vi "Write Rectifier Recipe to ListBox.vi"(4 "Right AmpMins":dbl[](array[numeric]), 5 "Left AmpMins":dbl[](array[numeric]), 6 "Right Amps":dbl[](array[numeric]), 7 "Left Amps":dbl[](array[numeric]), 8 "error in (no error)":errorcluster, 10 "Number Steps":i32, 11 "ListBox":refnum<vi>) -> (0 "error out":errorcluster)   [LabVIEW 2019]
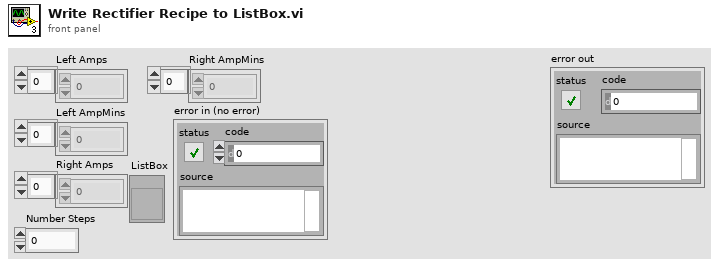
[diagram p1: front panel]
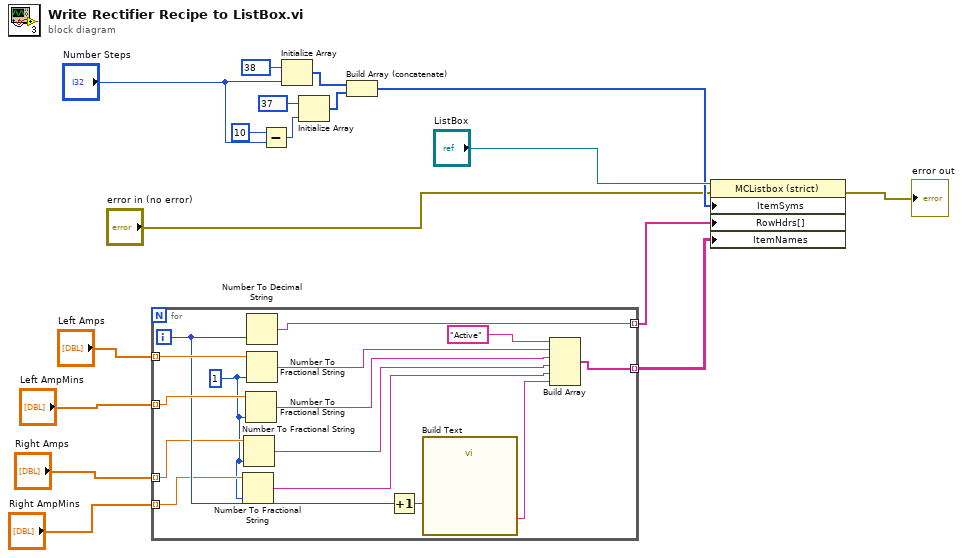
[diagram p0: block diagram]
diagram:
  n1 = for {
    tunnel: [w32] -> w2 mode=indexing
    tunnel: "Left Amps" -> [w29] mode=indexing
    tunnel: "Left AmpMins" -> [w26] mode=indexing
    tunnel: "Right Amps" -> [w23] mode=indexing
    tunnel: "Right AmpMins" -> [w21] mode=indexing
    tunnel: [w18] -> w1 mode=indexing
    i -> [w24]
    w20 = i16 1 ("precision (6)")
    n2 = Number To Fractional String(number=w21, precision (6)=w20) -> (F-format string=w19:string)  [unwired: 2 in]
    n3 = Number To Fractional String(number=w23, precision (6)=w20) -> (F-format string=w22:string)  [unwired: 2 in]
    n4 = Number To Fractional String(number=w26, precision (6)=w20) -> (F-format string=w25:string)  [unwired: 2 in]
    n5 = Number To Decimal String(number=w24) -> (decimal integer string=w32:string)  [unwired: 1 in]
    n6 = Number To Fractional String(number=w29, precision (6)=w20) -> (F-format string=w27:string)  [unwired: 2 in]
    n7 = Increment(x=w24) -> (x+1=w30:i32)
    n8 = call "Build Text"("d"=w30) -> ("Result"=w28:string)  [unwired: 13 in, 1 out]
    n9 = Build Array("Active", w27, w25, w22, w19, w28) -> (w18:string[])
  }
  n10 = Subtract(x=10, y="Number Steps") -> (x-y=w15:i32)
  n11 = Initialize Array(38, "Number Steps") -> (w14:i32[])
  n12 = Initialize Array(37, w15) -> (w13:i32[])
  n13 = Build Array (concatenate)(w14, w13) -> (w5:i32[])
  n14 = property class="MCListbox (strict)"(reference="ListBox", error in="error in (no error)", "ItemSyms"=w5, "RowHdrs[]"=w2, "ItemNames"=w1) -> (error out=→"error out":errorcluster)  [unwired: 1 out]
